vi "Combustion Model.vi"(8 "phi":sgl, 9 "Spark Advance (deg BTDC)":sgl, 10 "Engine Speed (rad/s)":sgl, 11 "Air Charge (g)":sgl) -> (2 "Torque (N-m)":sgl)   [LabVIEW 2016, in "NI-PCG Vehicle Model.lvlib"]
uses:
  NI-PCG Vehicle Model.lvlib
  Globals/Parameters.vi
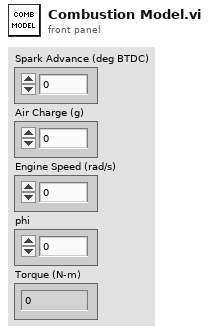
[diagram p1: front panel]
types:
  T1 = cluster{"Spark Timing (deg BTDC))":sgl[], "Engine Speed (RPM)":sgl[], "Combustion Efficiency":sgl[][]}
  T2 = typedef "NI-PCG Vehicle Model.lvlib/Engine Parameters.ctl" = cluster{"Ambient Parameters":cluster{"Temperature (K)":sgl, "Pressure (Pa)":sgl}, "Air Parameters":cluster{"R (Ideal Gas Constant)":sgl, "Molecular Weight":sgl, "Cp (Specific Heat Constant)":sgl, "Density (kg/m^3)":sgl, "Stoichiometric A/F Ratio":sgl}, "Engine Geometry Parameters":cluster{"Cylinder Volume (l)":sgl, "J (Rotational Moment of Inertia)":sgl, "Minimuim Engine Speed":sgl, "Maximum Engine Speed":sgl, "Intake Manifold Volume (l)":sgl}, "Volumetric Efficiency Map":cluster{"MAP":sgl[], "RPM":sgl[], "Table":sgl[][]}, "Fuel LHV (J/kg)":sgl, "Combustion Efficiency Map":cluster{"Spark Timing (deg BTDC))":sgl[], "Engine Speed (RPM)":sgl[], "Combustion Efficiency":sgl[][]}, "Thermodynamic Efficiency":sgl}
  T3 = typedef "NI-PCG Vehicle Model.lvlib/Transmission Parameters.ctl" = cluster{"Final Drive Ratio":sgl, "Transmission Gear Ratios":cluster{"Gears":sgl[], "Gear Ratios":sgl[]}, "Torque Converter Map":cluster{"Speed Ratio":sgl[], "K Factor":sgl[], "Torque Ratio":sgl[]}, "Upshift Throttle":sgl[], "Downshift Throttle":sgl[], "Upshift Table":sgl[][], "Downshift Table":sgl[][], "Wait Time":u8}
  T4 = typedef "NI-PCG Vehicle Model.lvlib/Vehicle Parameters.ctl" = cluster{"Vehicle Mass (kg)":sgl, "Vehicle Cd":sgl, "Vehicle Frontal Area (m^2)":sgl, "Wheel Radius (m)":sgl, "Wheel Rolling Resistance":sgl}
  T5 = cluster{"Engine Parameters":T2, "Transmission Parameters":T3, "Vehicle Parameters":T4}
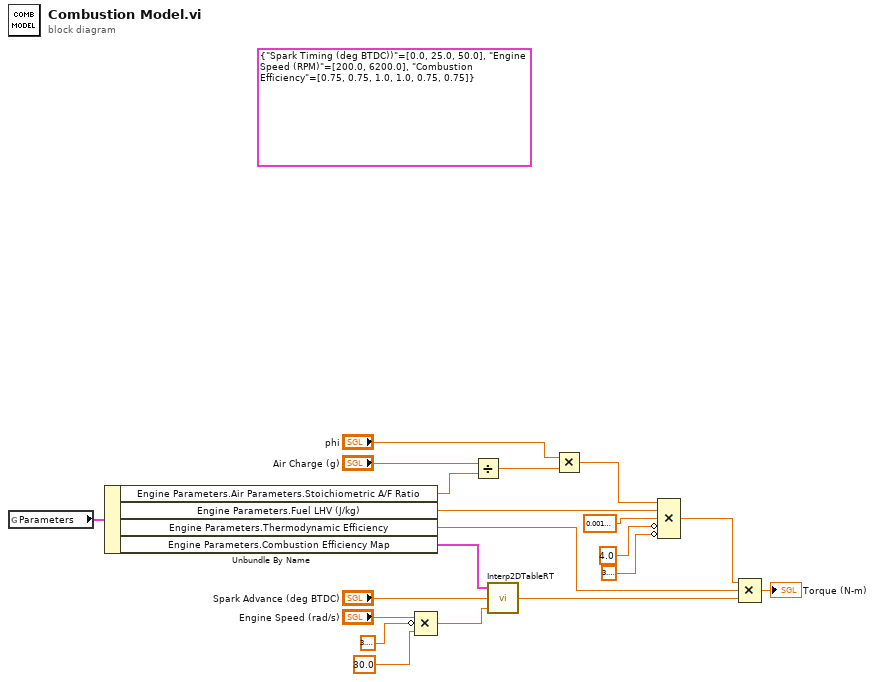
[diagram p0: block diagram]
diagram:
  (unwired) T1 {"Spark Timing (deg BTDC))"=[0.0, 25.0, 50.0], "Engine Speed (RPM)"=[200.0, 6200.0], "Combustion Efficiency"=[[0.75, 0.75], [1.0, 1.0], [0.75, 0.75]]} ("Combustion Efficiency Map")
  n1 = global read "Parameters.vi" "Parameters"() -> (w1:T5)
  n2 = Unbundle By Name(w1) -> ("Engine Parameters.Air Parameters.Stoichiometric A/F Ratio"=w20:sgl, "Engine Parameters.Fuel LHV (J/kg)"=w15:sgl, "Engine Parameters.Thermodynamic Efficiency"=w2:sgl, "Engine Parameters.Combustion Efficiency Map"=w4:T1)
  n3 = Compound Arithmetic op=MULTIPLY("Engine Speed (rad/s)", invert sgl 3.1415927, sgl 30.0 ("value")) -> (w7:sgl)
  n4 = Divide(x="Air Charge (g)", y=w20) -> (x/y=w17:sgl)
  n5 = call <vilib>:"Interp2DTableRT.vi"("Y"=w7, "X"="Spark Advance (deg BTDC)", "2DTable"=w4) -> ("Z"=w3:sgl)
  n6 = Multiply(x="phi", y=w17) -> (x*y=w18:sgl)
  n7 = Compound Arithmetic op=MULTIPLY(w18, w15, sgl 0.001 ("value"), invert sgl 4.0 ("value"), invert sgl 3.1415927) -> (w6:sgl)
  n8 = Compound Arithmetic op=MULTIPLY(w6, w2, w3) -> (→"Torque (N-m)":sgl)
